vi "Edit Config.vi"(8 "error in (no error)":errorcluster, 11 "Modbus in":refnum<class "Modbus.lvclass">) -> (0 "error out":errorcluster, 3 "Modbus out":refnum<class "Modbus.lvclass">)   [LabVIEW 2018, in "Modbus.lvclass"]
doc: "Modbus.lvclass:Edit Config.vi\n\nThis VI is used to edit the Modbus configuration parameters.\n\nInstrument Communication Module Version 1.0\nJanuary, 2018 Original Code Consulting David Thomson\n www.originalcode.com"
uses:
  Modbus.lvclass
  Modbus Config.ctl
  ICM Modbus Data Type.ctl
  ICM Class Editor State.ctl
  ICM Editor Command.ctl
  Modbus.lvclass/Modbus.ctl
panel:
  out "Serial Ports":i32[](array[numeric])
  in  "Check":bool
  in  "Flash Save":bool
  in  "Save":bool
  in  "Revert":bool
  in  "Modbus Config":T1={"Port"=0, "Modbus Server Name"="localhost", "Serial/Ethernet"=FALSE, "Baud Rate"=0, "Serial Type"=enum."RTU", "Unit ID"=0, "Parity"=0, "Input Channels"=[], "Swap Words?"=FALSE} {"Parity" items=["None", "Odd", "Even"]}
  # "Since this VI reads an array of numbers directly\nfrom the hardware (e.g. it does not read a string),\nthe \"No-op\" Parser should be used with it."
  # "Serial Parameters"
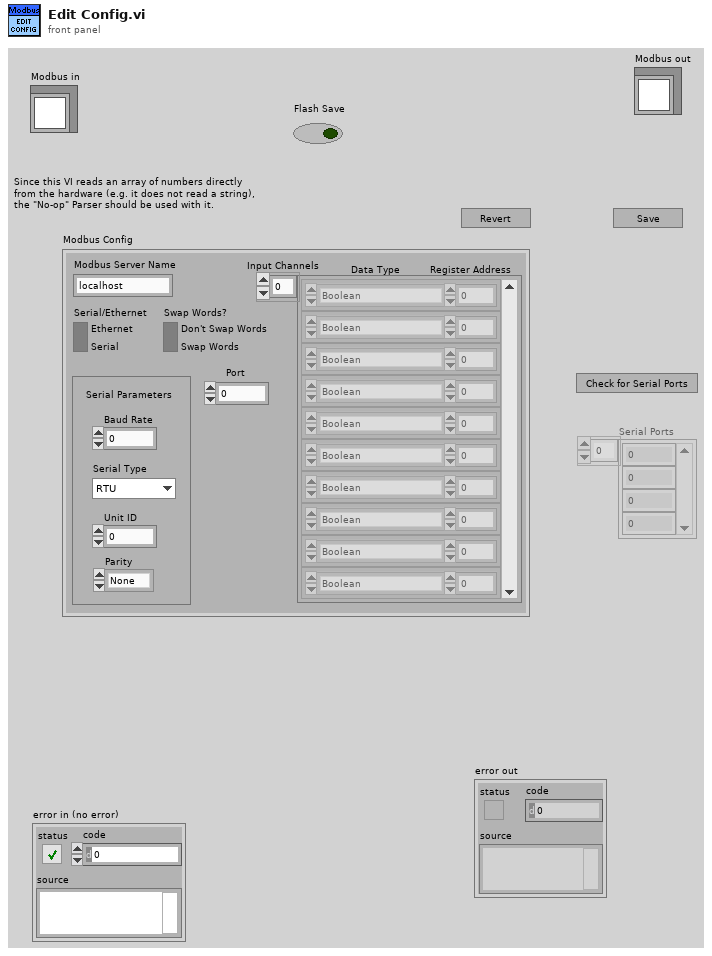
[diagram p1: front panel]
types:
  T1 = typedef "Modbus Config.ctl" = cluster{"Port":u16, "Modbus Server Name":string, "Serial/Ethernet":bool, "Baud Rate":u32, "Serial Type":enum16{"RTU", "ASCII"}, "Unit ID":u8, "Parity":u16, "Input Channels":cluster{"Data Type":T2, "Address":u16}[], "Swap Words?":bool}
  T2 = typedef "ICM Modbus Data Type.ctl" = enum16{"Boolean", "U16 (unsigned 16bit Int)", "I16 (signed 16bit Int)", "U32 (unsigned 32bit Int)", "I32 (signed 32bit Int)", "Real (Single 32bit)"}
  T3 = typedef "ICM Editor Command.ctl" = enum16{"No-op", "Exit"}
  T4 = typedef "ICM Class Editor State.ctl" = enum16{"Init", "Wait", "Write", "Read", "Display", "Set Flashing", "Error", "Stop"}
  T5 = enum8{"Enabled", "Disabled", "Disabled and Grayed Out"}
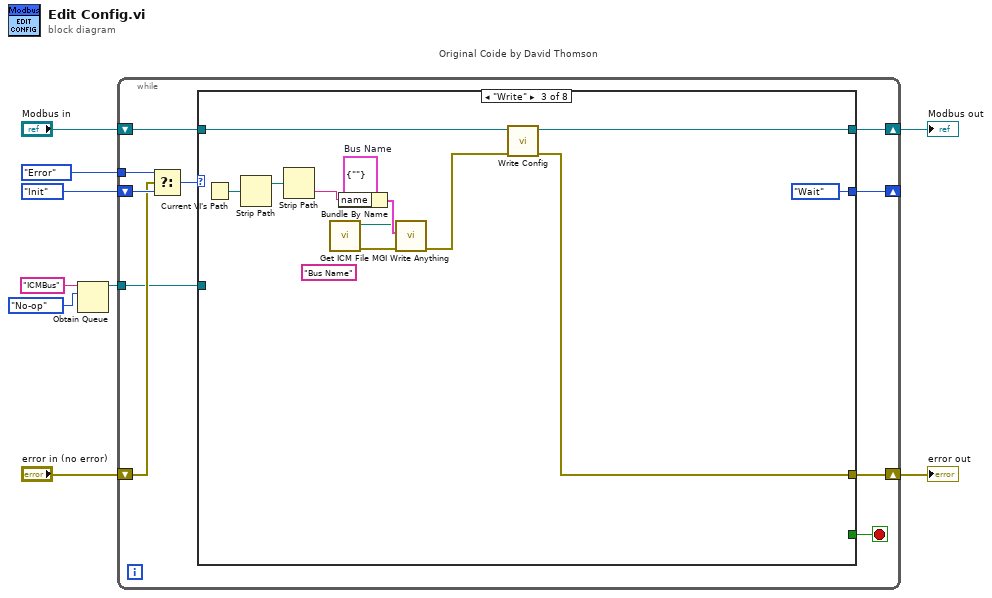
[diagram p0: block diagram]
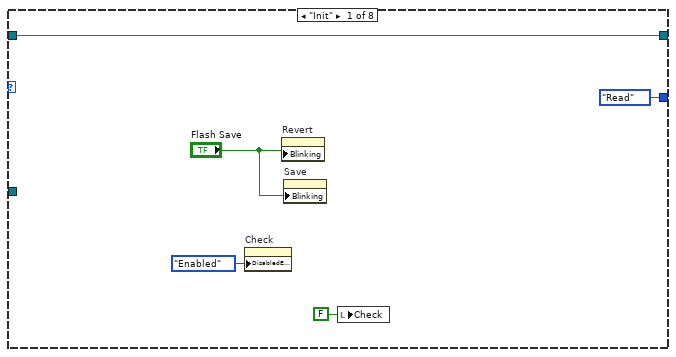
[diagram p2: hidden frame]
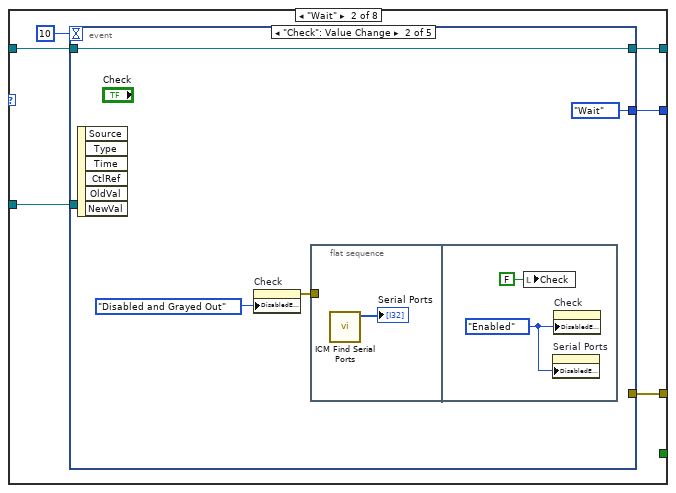
[diagram p3: hidden frame]
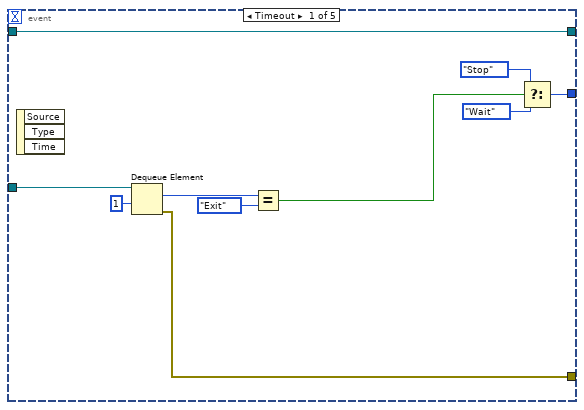
[diagram p4: hidden frame]
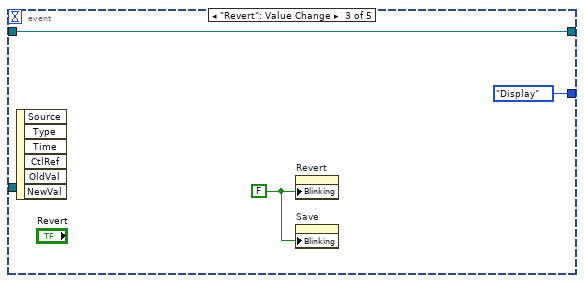
[diagram p5: hidden frame]
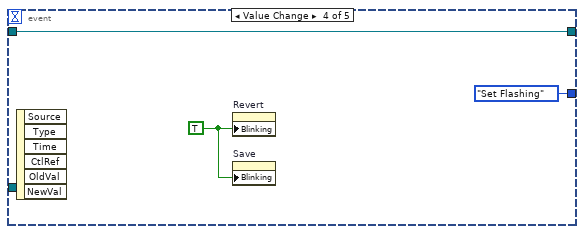
[diagram p6: hidden frame]
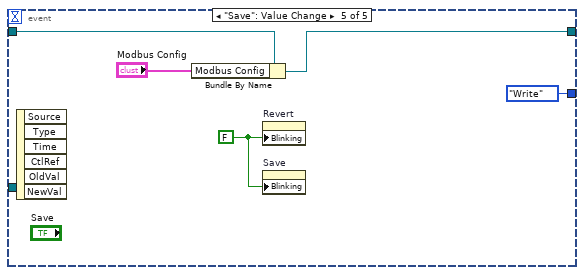
[diagram p7: hidden frame]
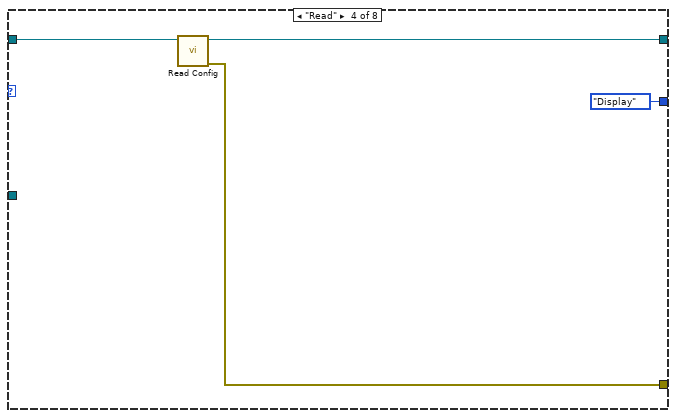
[diagram p8: hidden frame]
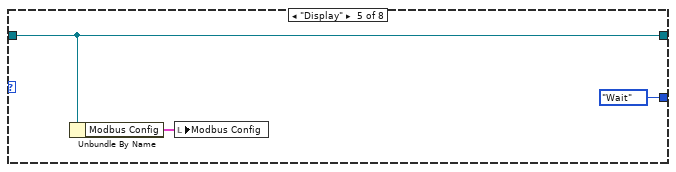
[diagram p9: hidden frame]
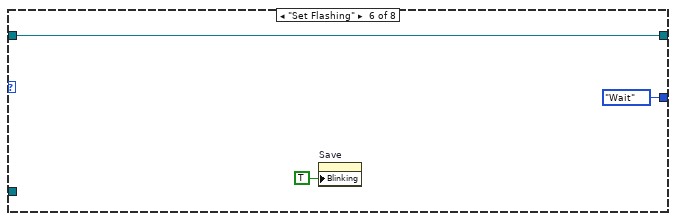
[diagram p10: hidden frame]
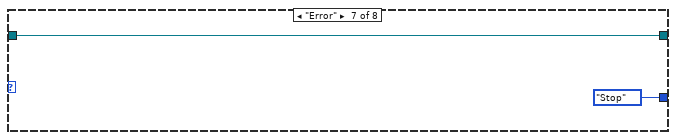
[diagram p11: hidden frame]
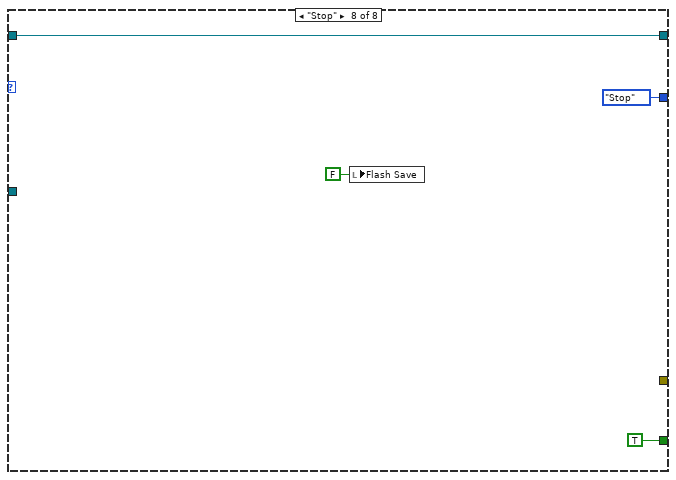
[diagram p12: hidden frame]
diagram:
  n1 = Obtain Queue(name (unnamed)="ICMBus", element data type=ICM_Editor_Command."No-op" ("Editor Command")) -> (queue out=w1:refnum<queue>)  [unwired: 3 in, 2 out]
  n2 = while "Original Coide by David Thomson" {
    shift-right: [w19] -> w8
    shift-left: "Modbus in" -> [w18]
    shift-right: [w12] -> _
    shift-left: ICM_Class_Editor_State."Init" ("Config State") -> [w16]
    shift-right: [w11] -> w6
    shift-left: "error in (no error)" -> [w14]
    tunnel: ICM_Class_Editor_State."Error" ("Config State") -> [w13]
    tunnel: w1 -> [w10]
    stop <- w17 stop-if-true
    n3 = Select(t=w13, s=w14, f=w16) -> (s? t:f=w15:T4)
    n4 = case shown="\"Write\"" w15 {
      tunnel: [w23 w28 w68 w72 w77 w80 w82 w86] -> w19
      tunnel: w18 -> [w23 w27 w69 w74 w77 w80 w82 w86]
      tunnel: [_ _ _ _ _ _ _ TRUE] -> w17
      tunnel: [ICM_Class_Editor_State."Read" ("Config State") w29 ICM_Class_Editor_State."Wait" ("Config State") ICM_Class_Editor_State."Display" ("Config State") ICM_Class_Editor_State."Wait" ("Config State") ICM_Class_Editor_State."Wait" ("Config State") ICM_Class_Editor_State."Stop" ("Config State") ICM_Class_Editor_State."Stop" ("Config State")] -> w12
      tunnel: [_ w25 w67 w73 _ _ _ _] -> w11
      tunnel: w10 -> [_ w26 _ _ _ _ _ _]
      frame "Init" {
        n5 = property on="Check" class="Bool (strict)"("DisabledEnum"=T5."Enabled" ("Disabled")) -> ()  [unwired: 2 in, 2 out]
        n6 = property on="Revert" class="Bool"("Blinking"="Flash Save") -> ()  [unwired: 2 in, 2 out]
        n7 = property on="Save" class="Bool"("Blinking"="Flash Save") -> ()  [unwired: 2 in, 2 out]
        n8 = local write "Check"(FALSE ("Check")) -> ()
      }
      frame "Wait" {
        n9 = event shown="[1] \"Check\": Value Change" {
          selector: _ -> [_ _ _ _ _]
          dyn-events: _ -> [_ _ _ _ _]
          timeout: 10 -> [_ _ _ _ _]
          tunnel: [w37 ICM_Class_Editor_State."Wait" ("Config State") ICM_Class_Editor_State."Display" ("Config State") ICM_Class_Editor_State."Set Flashing" ("Config State") ICM_Class_Editor_State."Write" ("Config State")] -> w29
          tunnel: [w40 w44 w49 w53 w55] -> w28
          tunnel: w27 -> [w40 w44 w49 w53 w56]
          tunnel: w26 -> [w39 _ _ _ _]
          tunnel: [w31 _ _ _ _] -> w25
          event Timeout {
            n10 = event-data() -> ()  [unwired: 1 in, 3 out]
            n11 = Dequeue Element(queue=w39, timeout in ms (-1)=1) -> (element=w36:T3, error out=w31:errorcluster)  [unwired: 1 in, 2 out]
            n12 = Equal?(x=w36, y=ICM_Editor_Command."Exit") -> (x = y?=w34:bool)
            n13 = Select(t=ICM_Class_Editor_State."Stop" ("Config State"), s=w34, f=ICM_Class_Editor_State."Wait" ("Config State")) -> (s? t:f=w37:T4)
          }
          event "Check": Value Change {
            n14 = event-data() -> ()  [unwired: 1 in, 6 out]
            n15 = property on="Check" class="Bool (strict)"("DisabledEnum"=T5."Disabled and Grayed Out" ("Disabled")) -> (error out=w42:errorcluster)  [unwired: 2 in, 1 out]
            n16 = flat-sequence {
              tunnel: w42 -> [_]
              frame #0 {
                n17 = call "ICM Find Serial Ports.vi"() -> ("Serial Ports"=→"Serial Ports":i32[])  [unwired: 11 in]
              }
              frame #1 {
                w46 = T5."Enabled" ("Disabled")
                n18 = local write "Check"(FALSE ("Check")) -> ()
                n19 = property on="Serial Ports" class="Arr (strict)"("DisabledEnum"=w46) -> ()  [unwired: 2 in, 2 out]
                n20 = property on="Check" class="Bool (strict)"("DisabledEnum"=w46) -> ()  [unwired: 2 in, 2 out]
              }
            }
          }
          event "Revert": Value Change {
            w48 = FALSE ("Blinking")
            n21 = event-data() -> ()  [unwired: 1 in, 6 out]
            n22 = property on="Revert" class="Bool"("Blinking"=w48) -> ()  [unwired: 2 in, 2 out]
            n23 = property on="Save" class="Bool"("Blinking"=w48) -> ()  [unwired: 2 in, 2 out]
          }
          event Value Change {
            w51 = TRUE ("Blinking")
            n24 = event-data() -> ()  [unwired: 1 in, 6 out]
            n25 = property on="Revert" class="Bool"("Blinking"=w51) -> ()  [unwired: 2 in, 2 out]
            n26 = property on="Save" class="Bool"("Blinking"=w51) -> ()  [unwired: 2 in, 2 out]
          }
          event "Save": Value Change {
            w54 = FALSE ("Blinking")
            n27 = event-data() -> ()  [unwired: 1 in, 6 out]
            n28 = Bundle By Name(cluster=w56, "Modbus Config"="Modbus Config") -> (w55:refnum<class "Modbus.lvclass">)
            n29 = property on="Revert" class="Bool"("Blinking"=w54) -> ()  [unwired: 2 in, 2 out]
            n30 = property on="Save" class="Bool"("Blinking"=w54) -> ()  [unwired: 2 in, 2 out]
          }
        }
      }
      frame "Write" {
        w63 = cluster{"name":string} {"name"=""}  # Bus Name
        (unwired) "Bus Name" ("Section Name (Name of \"Anything\")")
        n31 = Current VI's Path() -> (path=w66:path)
        n32 = Strip Path(path=w66) -> (stripped path=w65:path)  [unwired: 1 out]
        n33 = Strip Path(path=w65) -> (name=w62:string)  [unwired: 1 out]
        n34 = call "Get ICM File.vi"() -> ("error out"=w64:errorcluster, "ICM File"=w59:path)  [unwired: 10 in]
        n35 = Bundle By Name(cluster=w63, "name"=w62) -> (w61:cluster{"name":string})
        n36 = call "MGI Write Anything.vi"("Error In"=w64, "Anything"=w61, "Path (dialog)"=w59) -> ("Error Out"=w60:errorcluster)  [unwired: 6 in, 2 out]
        n37 = call-dynamic "Write Config.vi"("error in (no error)"=w60, "Modbus in"=w69) -> ("error out"=w67:errorcluster, "Modbus out"=w68:refnum<class "Modbus.lvclass">)  [unwired: 8 in]
      }
      frame "Read" {
        n38 = call-dynamic "Read Config.vi"("Modbus in"=w74) -> ("error out"=w73:errorcluster, "Modbus out"=w72:refnum<class "Modbus.lvclass">)  [unwired: 9 in]
      }
      frame "Display" {
        n39 = Unbundle By Name(w77) -> ("Modbus Config"=w76:T1)
        n40 = local write "Modbus Config"(w76) -> ()
      }
      frame "Set Flashing" {
        n41 = property on="Save" class="Bool"("Blinking"=TRUE) -> ()  [unwired: 2 in, 2 out]
      }
      frame "Error" {
      }
      frame "Stop" {
        n42 = local write "Flash Save"(FALSE ("Flash Save")) -> ()
      }
    }
  }
  "error out" <- w6
  "Modbus out" <- w8
